vi "Preferences.vi"(1 "Operation":enum16{"Load", "Save"}(ring)=enum."Save") -> ()   [LabVIEW 2013]
uses:
  Double Preference.vi
  Boolean Preference.vi
  PID Preference.vi
  <vilib>/Utility/config.llb/Read Key.vi
  <vilib>/Utility/config.llb/Read Key (Double).vi
  <vilib>/Rock Robotics/Network Tables/SD Write Number.vi
  <vilib>/Rock Robotics/Network Tables/SD Read Number.vi
  <vilib>/Utility/config.llb/Write Key.vi
  <vilib>/Utility/config.llb/Write Key (Double).vi
  <vilib>/Utility/config.llb/Read Key (Boolean).vi
  <vilib>/Rock Robotics/Network Tables/SD Write Boolean.vi
  <vilib>/Rock Robotics/Network Tables/SD Read Boolean.vi
  <vilib>/Utility/config.llb/Write Key (Boolean).vi
  <vilib>/Utility/config.llb/NI_LVConfig.lvlib
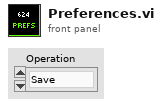
[diagram p1: front panel]
types:
  T1 = cluster{"high":dbl, "low":dbl, "P":dbl, "I":dbl, "D":dbl}
  T2 = typedef "NI_LVConfig.lvlib/Config Data RefNum.ctl" = refnum<k1>
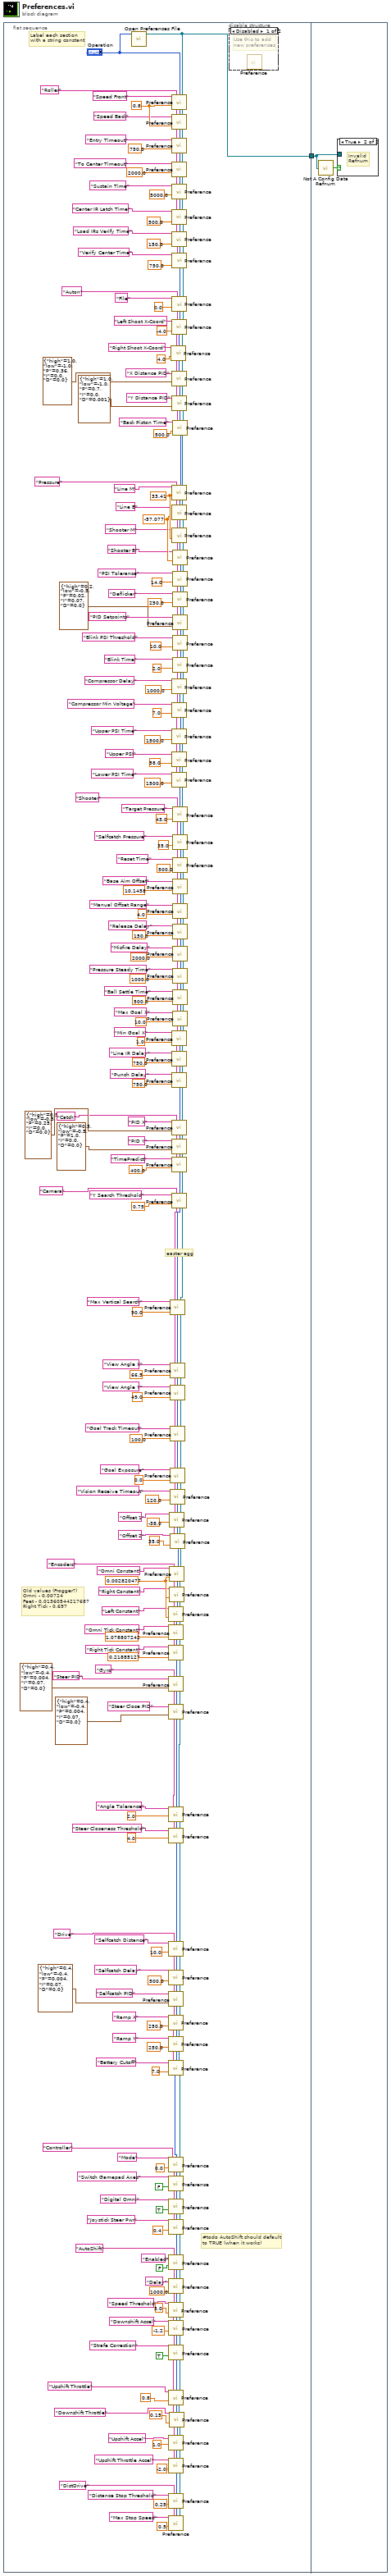
[diagram p0: block diagram]
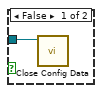
[diagram p3: hidden frame]
diagram:
  n1 = flat-sequence {
    tunnel: [w401] -> w1
    tunnel: w1 -> [w412]
    frame #0 {
      w153 = 0.002820477 ("default value")
      w216 = -57.077 ("default value")
      w219 = 33.41 ("default value")
      w405 = 0.8 ("default value")
      # "easter egg"
      # "#todo AutoShift should default\nto TRUE (when it works)"
      # "Old values (Frogger?)\nOmni - 0.00724\nFeet - 0.01360544217687\nRight Tick - 0.697"
      # "Label each section\nwith a string constant"
      n2 = call "Open Preferences File.vi"("Operation"="Operation") -> ("File refnum out"=w401:T2)  [unwired: 9 in, 1 out]
      n3 = call-poly "Preference.vi"("key"="Speed Front", "section"="Roller", "Operation"="Operation", "refnum in"=w401, "default value"=w405) -> ("section out"=w409:string, "Operation out"=w408:enum16{"Load", "Save"}, "refnum out"=w407:T2)  [unwired: 8 in]
      n4 = call-poly "Preference.vi"("key"="Speed Back", "section"=w409, "Operation"=w408, "refnum in"=w407, "default value"=w405) -> ("section out"=w395:string, "Operation out"=w397:enum16{"Load", "Save"}, "refnum out"=w396:T2)  [unwired: 8 in]
      n5 = call-poly "Preference.vi"("key"="Entry Timeout", "section"=w395, "Operation"=w397, "refnum in"=w396, "default value"=750.0) -> ("section out"=w398:string, "Operation out"=w400:enum16{"Load", "Save"}, "refnum out"=w399:T2)  [unwired: 8 in]
      n6 = call-poly "Preference.vi"("key"="To Center Timeout", "section"=w398, "Operation"=w400, "refnum in"=w399, "default value"=2000.0) -> ("section out"=w390:string, "Operation out"=w389:enum16{"Load", "Save"}, "refnum out"=w388:T2)  [unwired: 8 in]
      n7 = call-poly "Preference.vi"("key"="Sustain Time", "section"=w390, "Operation"=w389, "refnum in"=w388, "default value"=5000.0) -> ("section out"=w382:string, "Operation out"=w384:enum16{"Load", "Save"}, "refnum out"=w383:T2)  [unwired: 8 in]
      n8 = call-poly "Preference.vi"("key"="Center IR Latch Time", "section"=w382, "Operation"=w384, "refnum in"=w383, "default value"=500.0) -> ("section out"=w376:string, "Operation out"=w377:enum16{"Load", "Save"}, "refnum out"=w375:T2)  [unwired: 8 in]
      n9 = call-poly "Preference.vi"("key"="Load IRs Verify Time", "section"=w376, "Operation"=w377, "refnum in"=w375, "default value"=150.0) -> ("section out"=w57:string, "Operation out"=w56:enum16{"Load", "Save"}, "refnum out"=w55:T2)  [unwired: 8 in]
      n10 = call-poly "Preference.vi"("key"="Verify Center Time", "section"=w57, "Operation"=w56, "refnum in"=w55, "default value"=750.0) -> ("Operation out"=w54:enum16{"Load", "Save"}, "refnum out"=w53:T2)  [unwired: 8 in, 1 out]
      n11 = call-poly "Preference.vi"("key"="File", "section"="Auton", "Operation"=w54, "refnum in"=w53, "default value"=0.0) -> ("section out"=w365:string, "Operation out"=w366:enum16{"Load", "Save"}, "refnum out"=w367:T2)  [unwired: 8 in]
      n12 = call-poly "Preference.vi"("key"="Left Shoot X-Coord", "section"=w365, "Operation"=w366, "refnum in"=w367, "default value"=-4.0) -> ("section out"=w372:string, "Operation out"=w373:enum16{"Load", "Save"}, "refnum out"=w374:T2)  [unwired: 8 in]
      n13 = call-poly "Preference.vi"("key"="Right Shoot X-Coord", "section"=w372, "Operation"=w373, "refnum in"=w374, "default value"=4.0) -> ("section out"=w227:string, "Operation out"=w226:enum16{"Load", "Save"}, "refnum out"=w225:T2)  [unwired: 8 in]
      n14 = call-poly "Preference.vi"("key"="X Distance PID", "section"=w227, "Operation"=w226, "refnum in"=w225, "default value"=T1 {"high"=1.0, "low"=-1.0, "P"=0.36, "I"=0.0, "D"=0.0}) -> ("section out"=w230:string, "Operation out"=w229:enum16{"Load", "Save"}, "refnum out"=w228:T2)  [unwired: 8 in]
      n15 = call-poly "Preference.vi"("key"="Y Distance PID", "section"=w230, "Operation"=w229, "refnum in"=w228, "default value"=T1 {"high"=1.0, "low"=-1.0, "P"=0.7, "I"=0.0, "D"=0.001}) -> ("section out"=w60:string, "Operation out"=w64:enum16{"Load", "Save"}, "refnum out"=w61:T2)  [unwired: 8 in]
      n16 = call-poly "Preference.vi"("key"="Back Piston Time", "section"=w60, "Operation"=w64, "refnum in"=w61, "default value"=500.0) -> ("Operation out"=w63:enum16{"Load", "Save"}, "refnum out"=w62:T2)  [unwired: 8 in, 1 out]
      n17 = call-poly "Preference.vi"("key"="Line M", "section"="Pressure", "Operation"=w63, "refnum in"=w62, "default value"=w219) -> ("section out"=w233:string, "Operation out"=w232:enum16{"Load", "Save"}, "refnum out"=w231:T2)  [unwired: 8 in]
      n18 = call-poly "Preference.vi"("key"="Line B", "section"=w233, "Operation"=w232, "refnum in"=w231, "default value"=w216) -> ("section out"=w236:string, "Operation out"=w235:enum16{"Load", "Save"}, "refnum out"=w234:T2)  [unwired: 8 in]
      n19 = call-poly "Preference.vi"("key"="Shooter M", "section"=w236, "Operation"=w235, "refnum in"=w234, "default value"=w219) -> ("section out"=w239:string, "Operation out"=w238:enum16{"Load", "Save"}, "refnum out"=w237:T2)  [unwired: 8 in]
      n20 = call-poly "Preference.vi"("key"="Shooter B", "section"=w239, "Operation"=w238, "refnum in"=w237, "default value"=w216) -> ("section out"=w242:string, "Operation out"=w241:enum16{"Load", "Save"}, "refnum out"=w240:T2)  [unwired: 8 in]
      n21 = call-poly "Preference.vi"("key"="PSI Tolerance", "section"=w242, "Operation"=w241, "refnum in"=w240, "default value"=14.0) -> ("section out"=w245:string, "Operation out"=w244:enum16{"Load", "Save"}, "refnum out"=w243:T2)  [unwired: 8 in]
      n22 = call-poly "Preference.vi"("key"="Deflicker", "section"=w245, "Operation"=w244, "refnum in"=w243, "default value"=250.0) -> ("section out"=w248:string, "Operation out"=w247:enum16{"Load", "Save"}, "refnum out"=w246:T2)  [unwired: 8 in]
      n23 = call-poly "Preference.vi"("key"="PID Setpoints", "section"=w248, "Operation"=w247, "refnum in"=w246, "default value"=T1 {"high"=0.2, "low"=-0.5, "P"=0.02, "I"=0.07, "D"=0.0}) -> ("section out"=w251:string, "Operation out"=w250:enum16{"Load", "Save"}, "refnum out"=w249:T2)  [unwired: 8 in]
      n24 = call-poly "Preference.vi"("key"="Blink PSI Threshold", "section"=w251, "Operation"=w250, "refnum in"=w249, "default value"=10.0) -> ("section out"=w254:string, "Operation out"=w253:enum16{"Load", "Save"}, "refnum out"=w252:T2)  [unwired: 8 in]
      n25 = call-poly "Preference.vi"("key"="Blink Time", "section"=w254, "Operation"=w253, "refnum in"=w252, "default value"=2.0) -> ("section out"=w93:string, "Operation out"=w99:enum16{"Load", "Save"}, "refnum out"=w92:T2)  [unwired: 8 in]
      n26 = call-poly "Preference.vi"("key"="Compressor Delay", "section"=w93, "Operation"=w99, "refnum in"=w92, "default value"=1000.0) -> ("section out"=w96:string, "Operation out"=w95:enum16{"Load", "Save"}, "refnum out"=w94:T2)  [unwired: 8 in]
      n27 = call-poly "Preference.vi"("key"="Compressor Min Voltage", "section"=w96, "Operation"=w95, "refnum in"=w94, "default value"=7.0) -> ("section out"=w45:string, "Operation out"=w44:enum16{"Load", "Save"}, "refnum out"=w43:T2)  [unwired: 8 in]
      n28 = call-poly "Preference.vi"("key"="Upper PSI Time", "section"=w45, "Operation"=w44, "refnum in"=w43, "default value"=1500.0) -> ("section out"=w50:string, "Operation out"=w51:enum16{"Load", "Save"}, "refnum out"=w52:T2)  [unwired: 8 in]
      n29 = call-poly "Preference.vi"("key"="Upper PSI", "section"=w50, "Operation"=w51, "refnum in"=w52, "default value"=58.0) -> ("section out"=w40:string, "Operation out"=w39:enum16{"Load", "Save"}, "refnum out"=w38:T2)  [unwired: 8 in]
      n30 = call-poly "Preference.vi"("key"="Lower PSI Time", "section"=w40, "Operation"=w39, "refnum in"=w38, "default value"=1500.0) -> ("Operation out"=w37:enum16{"Load", "Save"}, "refnum out"=w36:T2)  [unwired: 8 in, 1 out]
      n31 = call-poly "Preference.vi"("key"="Target Pressure", "section"="Shooter", "Operation"=w37, "refnum in"=w36, "default value"=43.0) -> ("section out"=w257:string, "Operation out"=w256:enum16{"Load", "Save"}, "refnum out"=w255:T2)  [unwired: 8 in]
      n32 = call-poly "Preference.vi"("key"="Selfcatch Pressure", "section"=w257, "Operation"=w256, "refnum in"=w255, "default value"=35.0) -> ("section out"=w260:string, "Operation out"=w259:enum16{"Load", "Save"}, "refnum out"=w258:T2)  [unwired: 8 in]
      n33 = call-poly "Preference.vi"("key"="Reset Time" ("Name"), "section"=w260, "Operation"=w259, "refnum in"=w258, "default value"=500.0) -> ("section out"=w263:string, "Operation out"=w262:enum16{"Load", "Save"}, "refnum out"=w261:T2)  [unwired: 8 in]
      n34 = call-poly "Preference.vi"("key"="Base Aim Offset" ("Name"), "section"=w263, "Operation"=w262, "refnum in"=w261, "default value"=10.1458) -> ("section out"=w266:string, "Operation out"=w265:enum16{"Load", "Save"}, "refnum out"=w264:T2)  [unwired: 8 in]
      n35 = call-poly "Preference.vi"("key"="Manual Offset Range" ("Name"), "section"=w266, "Operation"=w265, "refnum in"=w264, "default value"=4.0) -> ("section out"=w269:string, "Operation out"=w268:enum16{"Load", "Save"}, "refnum out"=w267:T2)  [unwired: 8 in]
      n36 = call-poly "Preference.vi"("key"="Release Delay" ("Name"), "section"=w269, "Operation"=w268, "refnum in"=w267, "default value"=150.0) -> ("section out"=w272:string, "Operation out"=w271:enum16{"Load", "Save"}, "refnum out"=w270:T2)  [unwired: 8 in]
      n37 = call-poly "Preference.vi"("key"="Misfire Delay" ("Name"), "section"=w272, "Operation"=w271, "refnum in"=w270, "default value"=2000.0) -> ("section out"=w275:string, "Operation out"=w274:enum16{"Load", "Save"}, "refnum out"=w273:T2)  [unwired: 8 in]
      n38 = call-poly "Preference.vi"("key"="Pressure Steady Time" ("Name"), "section"=w275, "Operation"=w274, "refnum in"=w273, "default value"=1000.0) -> ("section out"=w278:string, "Operation out"=w277:enum16{"Load", "Save"}, "refnum out"=w276:T2)  [unwired: 8 in]
      n39 = call-poly "Preference.vi"("key"="Ball Settle Time" ("Name"), "section"=w278, "Operation"=w277, "refnum in"=w276, "default value"=500.0) -> ("section out"=w281:string, "Operation out"=w280:enum16{"Load", "Save"}, "refnum out"=w279:T2)  [unwired: 8 in]
      n40 = call-poly "Preference.vi"("key"="Max Goal X" ("Name"), "section"=w281, "Operation"=w280, "refnum in"=w279, "default value"=10.0) -> ("section out"=w284:string, "Operation out"=w283:enum16{"Load", "Save"}, "refnum out"=w282:T2)  [unwired: 8 in]
      n41 = call-poly "Preference.vi"("key"="Min Goal X" ("Name"), "section"=w284, "Operation"=w283, "refnum in"=w282, "default value"=1.0) -> ("section out"=w87:string, "Operation out"=w89:enum16{"Load", "Save"}, "refnum out"=w88:T2)  [unwired: 8 in]
      n42 = call-poly "Preference.vi"("key"="Line IR Delay" ("Name"), "section"=w87, "Operation"=w89, "refnum in"=w88, "default value"=750.0) -> ("section out"=w29:string, "Operation out"=w33:enum16{"Load", "Save"}, "refnum out"=w30:T2)  [unwired: 8 in]
      n43 = call-poly "Preference.vi"("key"="Punch Delay" ("Name"), "section"=w29, "Operation"=w33, "refnum in"=w30, "default value"=750.0) -> ("Operation out"=w32:enum16{"Load", "Save"}, "refnum out"=w31:T2)  [unwired: 8 in, 1 out]
      n44 = call-poly "Preference.vi"("key"="PID X", "section"="Catch", "Operation"=w32, "refnum in"=w31, "default value"=T1 {"high"=0.5, "low"=-0.5, "P"=0.25, "I"=0.0, "D"=0.0}) -> ("section out"=w287:string, "Operation out"=w286:enum16{"Load", "Save"}, "refnum out"=w285:T2)  [unwired: 8 in]
      n45 = call-poly "Preference.vi"("key"="PID Y", "section"=w287, "Operation"=w286, "refnum in"=w285, "default value"=T1 {"high"=0.5, "low"=-0.5, "P"=1.0, "I"=0.0, "D"=0.0}) -> ("section out"=w290:string, "Operation out"=w289:enum16{"Load", "Save"}, "refnum out"=w288:T2)  [unwired: 8 in]
      n46 = call-poly "Preference.vi"("key"="TimePredict", "section"=w290, "Operation"=w289, "refnum in"=w288, "default value"=400.0) -> ("Operation out"=w292:enum16{"Load", "Save"}, "refnum out"=w291:T2)  [unwired: 8 in, 1 out]
      n47 = call-poly "Preference.vi"("key"="Y Search Threshold", "section"="Camera", "Operation"=w292, "refnum in"=w291, "default value"=0.75) -> ("section out"=w5:string, "Operation out"=w6:enum16{"Load", "Save"}, "refnum out"=w7:T2)  [unwired: 8 in]
      n48 = call-poly "Preference.vi"("key"="Max Vertical Search", "section"=w5, "Operation"=w6, "refnum in"=w7, "default value"=90.0) -> ("section out"=w8:string, "Operation out"=w9:enum16{"Load", "Save"}, "refnum out"=w10:T2)  [unwired: 8 in]
      n49 = call-poly "Preference.vi"("key"="View Angle X", "section"=w8, "Operation"=w9, "refnum in"=w10, "default value"=66.5) -> ("section out"=w295:string, "Operation out"=w294:enum16{"Load", "Save"}, "refnum out"=w293:T2)  [unwired: 8 in]
      n50 = call-poly "Preference.vi"("key"="View Angle Y", "section"=w295, "Operation"=w294, "refnum in"=w293, "default value"=49.0) -> ("section out"=w13:string, "Operation out"=w12:enum16{"Load", "Save"}, "refnum out"=w11:T2)  [unwired: 8 in]
      n51 = call-poly "Preference.vi"("key"="Goal Track Timeout", "section"=w13, "Operation"=w12, "refnum in"=w11, "default value"=100.0) -> ("section out"=w14:string, "Operation out"=w15:enum16{"Load", "Save"}, "refnum out"=w16:T2)  [unwired: 8 in]
      n52 = call-poly "Preference.vi"("key"="Goal Exposure", "section"=w14, "Operation"=w15, "refnum in"=w16, "default value"=0.0) -> ("section out"=w298:string, "Operation out"=w297:enum16{"Load", "Save"}, "refnum out"=w296:T2)  [unwired: 8 in]
      n53 = call-poly "Preference.vi"("key"="Vision Receive Timeout", "section"=w298, "Operation"=w297, "refnum in"=w296, "default value"=120.0) -> ("section out"=w301:string, "Operation out"=w300:enum16{"Load", "Save"}, "refnum out"=w299:T2)  [unwired: 8 in]
      n54 = call-poly "Preference.vi"("key"="Offset 1", "section"=w301, "Operation"=w300, "refnum in"=w299, "default value"=-38.0) -> ("section out"=w304:string, "Operation out"=w303:enum16{"Load", "Save"}, "refnum out"=w302:T2)  [unwired: 8 in]
      n55 = call-poly "Preference.vi"("key"="Offset 2", "section"=w304, "Operation"=w303, "refnum in"=w302, "default value"=35.0) -> ("Operation out"=w306:enum16{"Load", "Save"}, "refnum out"=w305:T2)  [unwired: 8 in, 1 out]
      n56 = call-poly "Preference.vi"("key"="Omni Constant", "section"="Encoders" ("key"), "Operation"=w306, "refnum in"=w305, "default value"=w153) -> ("section out"=w309:string, "Operation out"=w308:enum16{"Load", "Save"}, "refnum out"=w307:T2)  [unwired: 8 in]
      n57 = call-poly "Preference.vi"("key"="Right Constant", "section"=w309, "Operation"=w308, "refnum in"=w307, "default value"=w153) -> ("section out"=w312:string, "Operation out"=w311:enum16{"Load", "Save"}, "refnum out"=w310:T2)  [unwired: 8 in]
      n58 = call-poly "Preference.vi"("key"="Left Constant", "section"=w312, "Operation"=w311, "refnum in"=w310, "default value"=w153) -> ("section out"=w315:string, "Operation out"=w314:enum16{"Load", "Save"}, "refnum out"=w313:T2)  [unwired: 8 in]
      n59 = call-poly "Preference.vi"("key"="Omni Tick Constant", "section"=w315, "Operation"=w314, "refnum in"=w313, "default value"=1.078807242) -> ("section out"=w318:string, "Operation out"=w317:enum16{"Load", "Save"}, "refnum out"=w316:T2)  [unwired: 8 in]
      n60 = call-poly "Preference.vi"("key"="Right Tick Constant", "section"=w318, "Operation"=w317, "refnum in"=w316, "default value"=0.21885127) -> ("Operation out"=w320:enum16{"Load", "Save"}, "refnum out"=w319:T2)  [unwired: 8 in, 1 out]
      n61 = call-poly "Preference.vi"("key"="Steer PID", "section"="Gyro", "Operation"=w320, "refnum in"=w319, "default value"=T1 {"high"=0.4, "low"=-0.4, "P"=0.004, "I"=0.07, "D"=0.0}) -> ("section out"=w85:string, "Operation out"=w84:enum16{"Load", "Save"}, "refnum out"=w83:T2)  [unwired: 8 in]
      n62 = call-poly "Preference.vi"("key"="Steer Close PID", "section"=w85, "Operation"=w84, "refnum in"=w83, "default value"=T1 {"high"=0.4, "low"=-0.4, "P"=0.004, "I"=0.07, "D"=0.0}) -> ("section out"=w2:string, "Operation out"=w3:enum16{"Load", "Save"}, "refnum out"=w4:T2)  [unwired: 8 in]
      n63 = call-poly "Preference.vi"("key"="Angle Tolerance", "section"=w2, "Operation"=w3, "refnum in"=w4, "default value"=2.0) -> ("section out"=w77:string, "Operation out"=w79:enum16{"Load", "Save"}, "refnum out"=w78:T2)  [unwired: 8 in]
      n64 = call-poly "Preference.vi"("key"="Steer Closeness Threshold", "section"=w77, "Operation"=w79, "refnum in"=w78, "default value"=4.0) -> ("Operation out"=w17:enum16{"Load", "Save"}, "refnum out"=w18:T2)  [unwired: 8 in, 1 out]
      n65 = call-poly "Preference.vi"("key"="Selfcatch Distance", "section"="Drive", "Operation"=w17, "refnum in"=w18, "default value"=10.0) -> ("section out"=w323:string, "Operation out"=w322:enum16{"Load", "Save"}, "refnum out"=w321:T2)  [unwired: 8 in]
      n66 = call-poly "Preference.vi"("key"="Selfcatch Delay", "section"=w323, "Operation"=w322, "refnum in"=w321, "default value"=500.0) -> ("section out"=w326:string, "Operation out"=w325:enum16{"Load", "Save"}, "refnum out"=w324:T2)  [unwired: 8 in]
      n67 = call-poly "Preference.vi"("key"="Selfcatch PID", "section"=w326, "Operation"=w325, "refnum in"=w324, "default value"=T1 {"high"=0.4, "low"=-0.4, "P"=0.004, "I"=0.07, "D"=0.0}) -> ("section out"=w329:string, "Operation out"=w328:enum16{"Load", "Save"}, "refnum out"=w327:T2)  [unwired: 8 in]
      n68 = call-poly "Preference.vi"("key"="Ramp X", "section"=w329, "Operation"=w328, "refnum in"=w327, "default value"=250.0) -> ("section out"=w332:string, "Operation out"=w331:enum16{"Load", "Save"}, "refnum out"=w330:T2)  [unwired: 8 in]
      n69 = call-poly "Preference.vi"("key"="Ramp Y", "section"=w332, "Operation"=w331, "refnum in"=w330, "default value"=250.0) -> ("section out"=w335:string, "Operation out"=w334:enum16{"Load", "Save"}, "refnum out"=w333:T2)  [unwired: 8 in]
      n70 = call-poly "Preference.vi"("key"="Battery Cutoff", "section"=w335, "Operation"=w334, "refnum in"=w333, "default value"=7.0) -> ("Operation out"=w19:enum16{"Load", "Save"}, "refnum out"=w20:T2)  [unwired: 8 in, 1 out]
      n71 = call-poly "Preference.vi"("key"="Mode", "section"="Controller", "Operation"=w19, "refnum in"=w20, "default value"=0.0) -> ("section out"=w338:string, "Operation out"=w337:enum16{"Load", "Save"}, "refnum out"=w336:T2)  [unwired: 8 in]
      n72 = call-poly "Preference.vi"("key"="Switch Gamepad Axes", "section"=w338, "Operation"=w337, "refnum in"=w336, "default value"=FALSE) -> ("section out"=w341:string, "Operation out"=w340:enum16{"Load", "Save"}, "refnum out"=w339:T2)  [unwired: 8 in]
      n73 = call-poly "Preference.vi"("key"="Digital Omni", "section"=w341, "Operation"=w340, "refnum in"=w339, "default value"=TRUE) -> ("section out"=w344:string, "Operation out"=w343:enum16{"Load", "Save"}, "refnum out"=w342:T2)  [unwired: 8 in]
      n74 = call-poly "Preference.vi"("key"="Joystick Steer Pwr", "section"=w344, "Operation"=w343, "refnum in"=w342, "default value"=0.4) -> ("Operation out"=w346:enum16{"Load", "Save"}, "refnum out"=w345:T2)  [unwired: 8 in, 1 out]
      n75 = call-poly "Preference.vi"("key"="Enabled", "section"="AutoShift", "Operation"=w346, "refnum in"=w345, "default value"=FALSE) -> ("section out"=w349:string, "Operation out"=w348:enum16{"Load", "Save"}, "refnum out"=w347:T2)  [unwired: 8 in]
      n76 = call-poly "Preference.vi"("key"="Delay", "section"=w349, "Operation"=w348, "refnum in"=w347, "default value"=1000.0) -> ("section out"=w352:string, "Operation out"=w351:enum16{"Load", "Save"}, "refnum out"=w350:T2)  [unwired: 8 in]
      n77 = call-poly "Preference.vi"("key"="Speed Threshold", "section"=w352, "Operation"=w351, "refnum in"=w350, "default value"=5.0) -> ("section out"=w355:string, "Operation out"=w354:enum16{"Load", "Save"}, "refnum out"=w353:T2)  [unwired: 8 in]
      n78 = call-poly "Preference.vi"("key"="Downshift Accel" ("Name"), "section"=w355, "Operation"=w354, "refnum in"=w353, "default value"=-1.2) -> ("section out"=w27:string, "Operation out"=w26:enum16{"Load", "Save"}, "refnum out"=w25:T2)  [unwired: 8 in]
      n79 = call-poly "Preference.vi"("key"="Strafe Correction", "section"=w27, "Operation"=w26, "refnum in"=w25, "default value"=TRUE) -> ("section out"=w21:string, "Operation out"=w24:enum16{"Load", "Save"}, "refnum out"=w23:T2)  [unwired: 8 in]
      n80 = call-poly "Preference.vi"("key"="Upshift Throttle" ("Name"), "section"=w21, "Operation"=w24, "refnum in"=w23, "default value"=0.8) -> ("section out"=w358:string, "Operation out"=w357:enum16{"Load", "Save"}, "refnum out"=w356:T2)  [unwired: 8 in]
      n81 = call-poly "Preference.vi"("key"="Downshift Throttle" ("Name"), "section"=w358, "Operation"=w357, "refnum in"=w356, "default value"=0.15) -> ("section out"=w361:string, "Operation out"=w360:enum16{"Load", "Save"}, "refnum out"=w359:T2)  [unwired: 8 in]
      n82 = call-poly "Preference.vi"("key"="Upshift Accel" ("Name"), "section"=w361, "Operation"=w360, "refnum in"=w359, "default value"=1.0) -> ("section out"=w364:string, "Operation out"=w363:enum16{"Load", "Save"}, "refnum out"=w362:T2)  [unwired: 8 in]
      n83 = call-poly "Preference.vi"("key"="Upshift Throttle Accel" ("Name"), "section"=w364, "Operation"=w363, "refnum in"=w362, "default value"=-2.0) -> ("Operation out"=w75:enum16{"Load", "Save"}, "refnum out"=w67:T2)  [unwired: 8 in, 1 out]
      n84 = call-poly "Preference.vi"("key"="Distance Stop Threshold" ("Name"), "section"="DistDrive" ("Name"), "Operation"=w75, "refnum in"=w67, "default value"=0.25) -> ("section out"=w69:string, "Operation out"=w70:enum16{"Load", "Save"}, "refnum out"=w68:T2)  [unwired: 8 in]
      n85 = call-poly "Preference.vi"("key"="Max Stop Speed" ("Name"), "section"=w69, "Operation"=w70, "refnum in"=w68, "default value"=0.5) -> ()  [unwired: 8 in, 3 out]
      n86 = disable-structure shown="Disabled" {
        frame Disabled {
          # "Use this to add\nnew preferences"
          n87 = call-poly "Preference.vi"() -> ()  [unwired: 13 in, 3 out]
        }
        frame Enabled {
        }
      }
    }
    frame #1 {
      n88 = call <vilib>:"Not A Config Data Refnum.vi"("refnum"=w412) -> ("not a config data refnum"=w413:bool)
      n89 = case shown="True" w413 {
        tunnel: w412 -> [w414 _]
        frame False {
          n90 = call <vilib>:"Close Config Data.vi"("refnum"=w414) -> ()  [unwired: 9 in, 2 out]
        }
        frame True {
          # "Invalid\nRefnum"
        }
      }
    }
  }
